vi "Parameters_file.vi"(0 "Record":bool, 1 "File location":path, 2 "actual sample rate array":dbl[](array[numeric]), 3 "actualSamples array":i32[](array[numeric]), 4 "Files name array":string[](array[string]), 5 "Additional text":string) -> (6 "Full text":string)   [LabVIEW 2011]
panel:
  in  "Explications":string
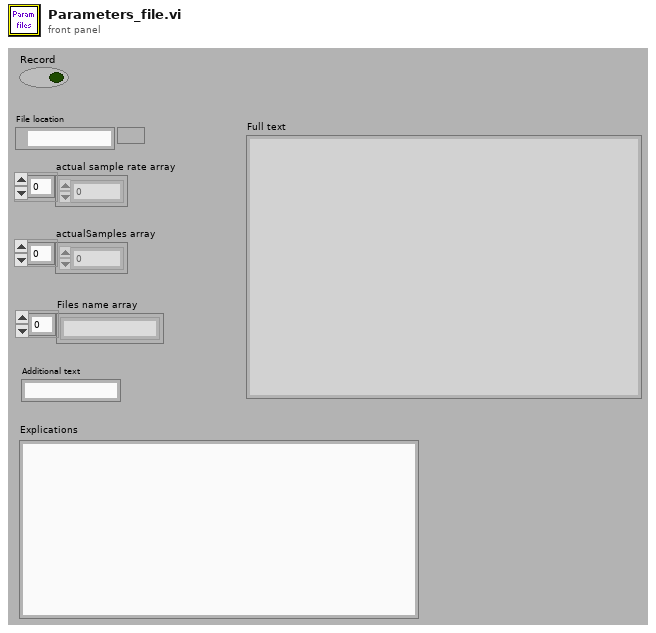
[diagram p1: front panel]
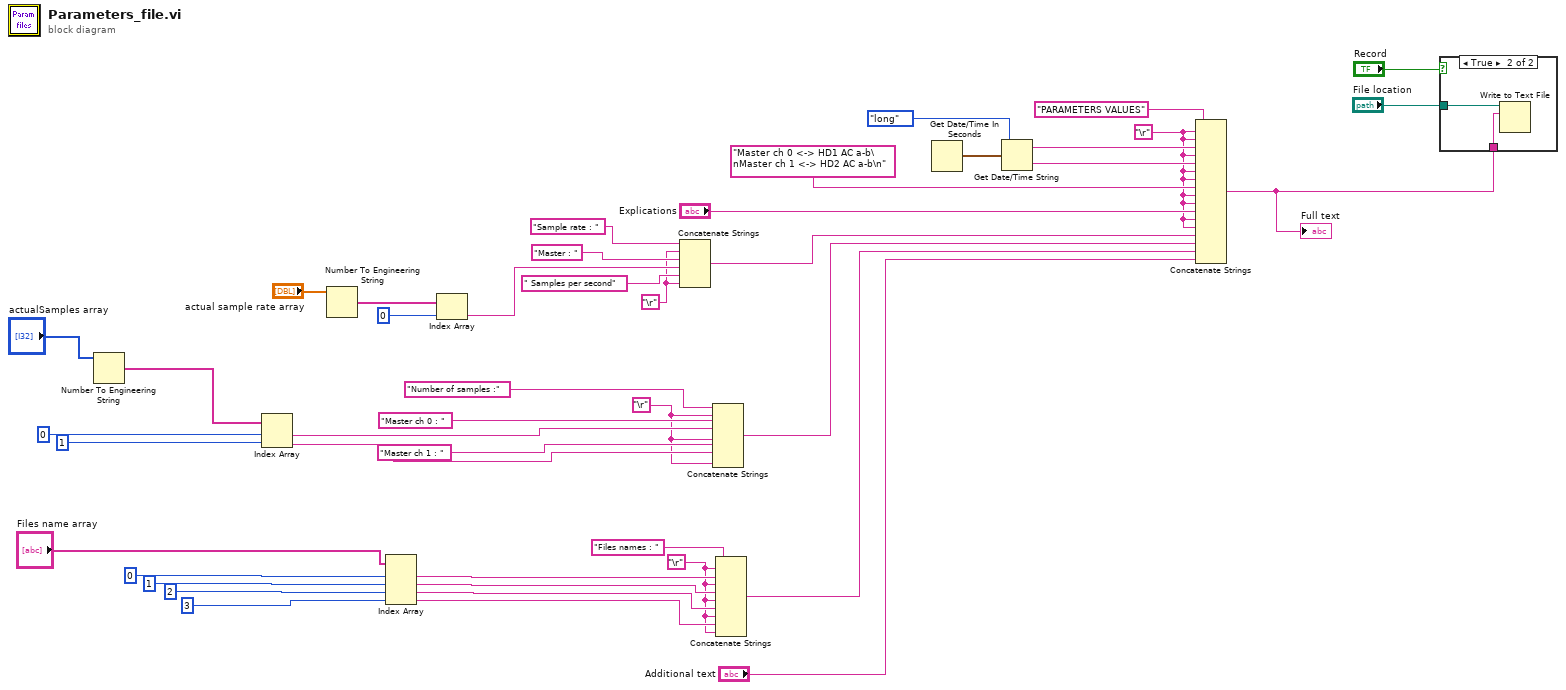
[diagram p0: block diagram]
diagram:
  w13 = "\r"
  w11 = "\r"
  w1 = "\r"
  w24 = "\r"
  n1 = Number To Engineering String(4:"actualSamples array") -> (0:w34:string[])  [unwired: 3 out]
  n2 = Index Array(array=w34, index #1=0 ("index"), index #2=1 ("index")) -> (element #1=w28:string, element #2=w26:string)
  n3 = Number To Engineering String(4:"actual sample rate array") -> (0:w18:string[])  [unwired: 3 out]
  n4 = Index Array(array="Files name array", index #1=0 ("index"), index #2=1 ("index"), index #3=2 ("index"), index #4=3 ("index")) -> (element #1=w6:string, element #2=w5:string, element #3=w4:string, element #4=w2:string)
  n5 = Index Array(array=w18, index=0) -> (element=w15:string)
  n6 = Concatenate Strings("Sample rate : " ("string"), w13, "Master : " ("string"), w15, " Samples per second" ("string"), w13) -> (w23:string)
  n7 = Concatenate Strings("Number of samples :" ("string"), w11, "Master ch 0 : " ("string"), w28, w11, "Master ch 1 : " ("string"), w26, w11) -> (w22:string)
  n8 = Concatenate Strings("Files names : " ("string"), w1, w6, w1, w5, w1, w4, w1, w2, w1) -> (w21:string)
  n9 = Get Date/Time In Seconds() -> (seconds since 1Jan1904=w41:timestamp)
  n10 = Get Date/Time String(date format (0)=enum16{"short", "long", "abbreviated"}."long", seconds (now)=w41) -> (date string=w38:string, time string=w40:string)  [unwired: 1 out]
  n11 = Concatenate Strings("PARAMETERS VALUES" ("string"), w24, w24, w38, w24, w40, w24, w24, "Master ch 0 <-> HD1 AC a-b\nMaster ch 1 <-> HD2 AC a-b\n", w24, w24, "Explications", w24, w24, w23, w22, w21, "Additional text") -> (w42:string)
  "Full text" <- w42
  n12 = case shown="True" "Record" {
    tunnel: "File location" -> [_ w46]
    tunnel: w42 -> [_ w45]
    frame False {
    }
    frame True {
      n13 = Write to Text File(file (use dialog)=w46, text=w45) -> ()  [unwired: 1 in, 4 out]
    }
  }
